vi "SVA 4MV6 T003 CCE.vi"() -> ()   [LabVIEW 2020]
panel:
  out "RGB":picture
  # "CEBALLOS CONDE  EMANUEL"
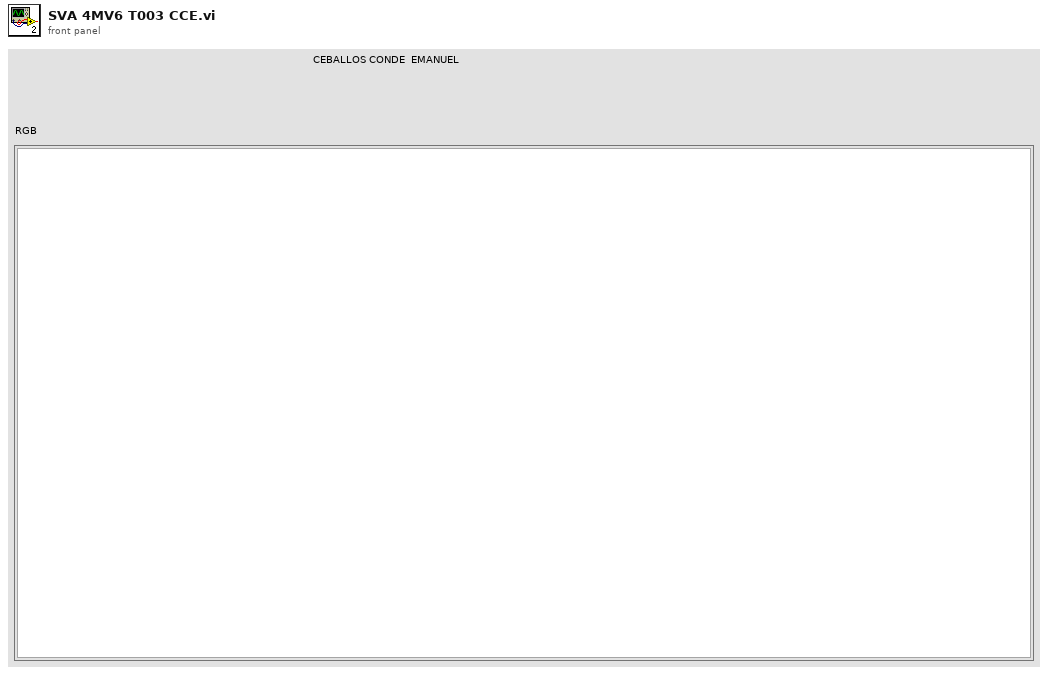
[diagram p1: front panel]
types:
  T1 = typedef "imagedata.ctl" = cluster{"image type":i32, "image depth":i32, "image":u8[], "mask":u8[], "colors":u32[], "Rectangle":cluster{"left":i16, "top":i16, "right":i16, "bottom":i16}}
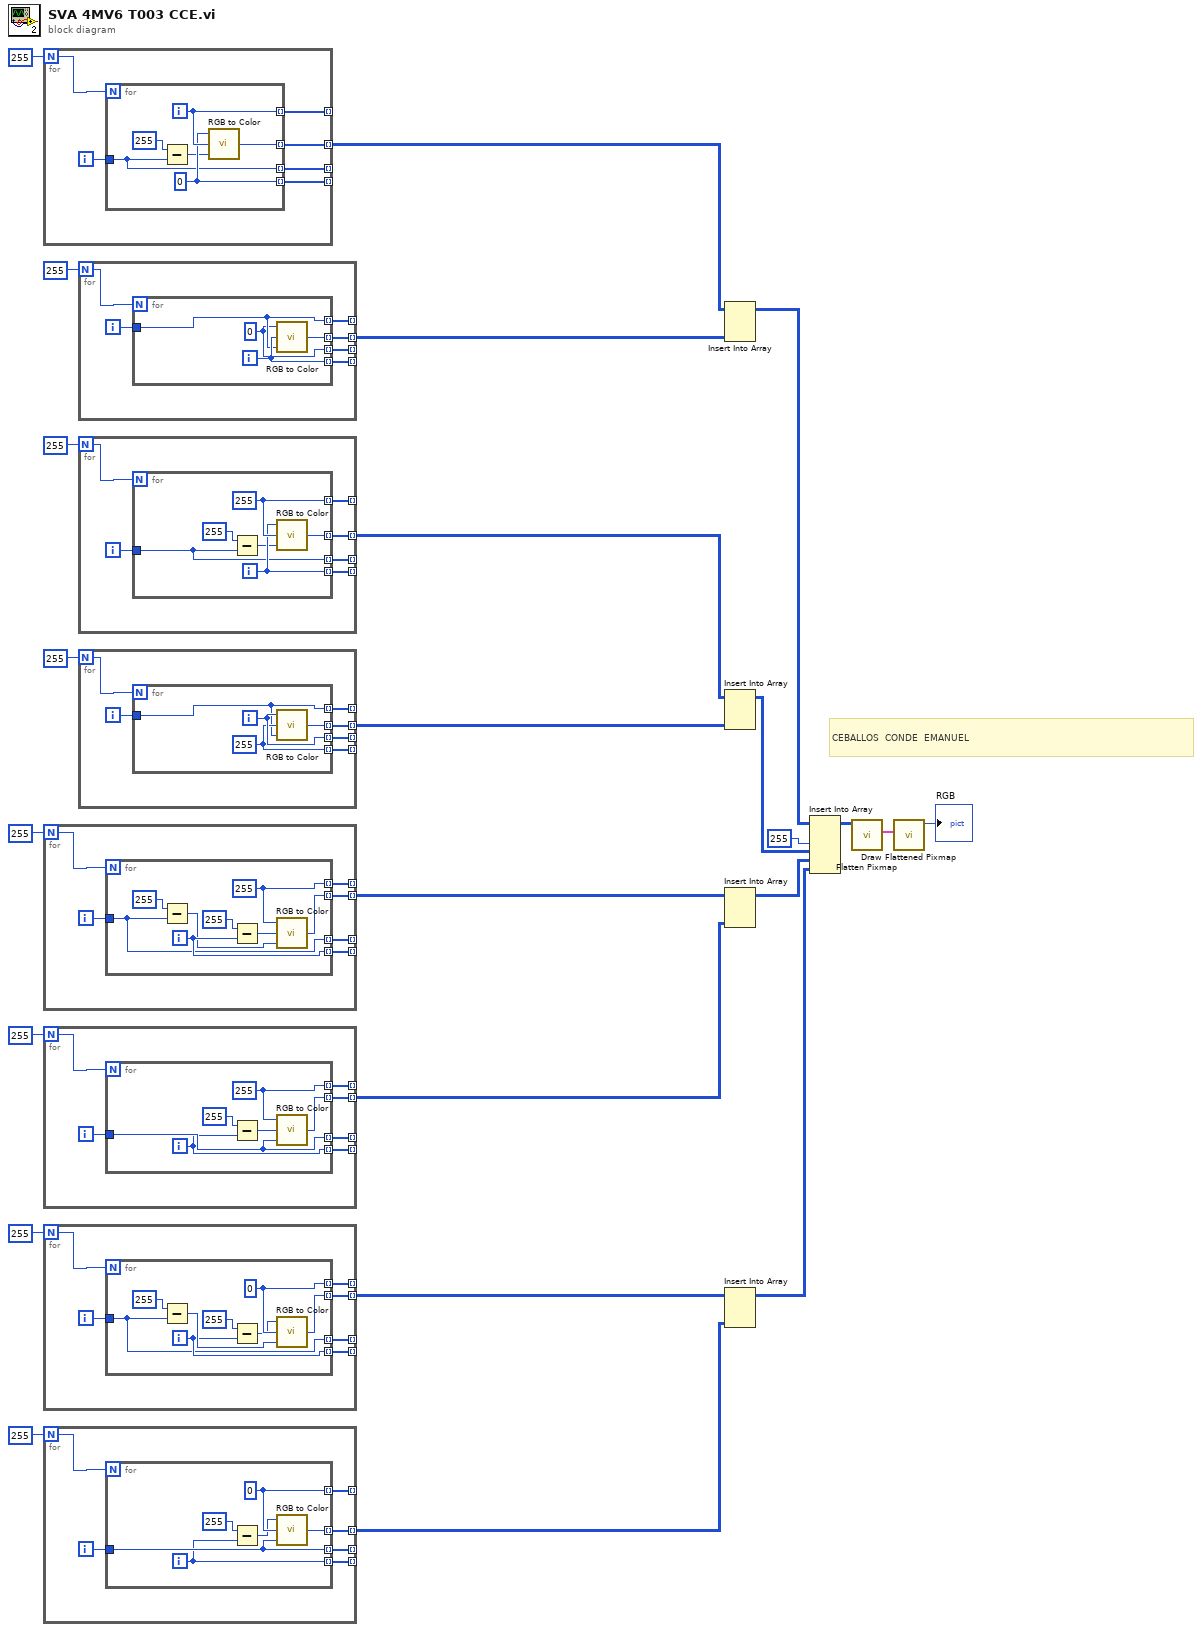
[diagram p0: block diagram]
diagram:
  # "CEBALLOS  CONDE  EMANUEL"
  n1 = for {
    N: 255 -> [w26]
    tunnel: [w30] -> _ mode=indexing
    tunnel: [w28] -> _ mode=indexing
    tunnel: [w27] -> _ mode=indexing
    tunnel: [w25] -> w4 mode=indexing
    i -> [w29]
    n2 = for {
      N: w26 -> [_]
      tunnel: [w35] -> w30 mode=indexing
      tunnel: w29 -> [w31]
      tunnel: [w31] -> w28 mode=indexing
      tunnel: [w34] -> w27 mode=indexing
      tunnel: [w36] -> w25 mode=indexing
      i -> [w35]
      w34 = 0
      n3 = Subtract(x=255, y=w31) -> (x-y=w32:i32)
      n4 = call <vilib>:"RGB to Color.vi"("B"=w32, "G"=w35, "R"=w34) -> ("Color"=w36:u32)
    }
  }
  n5 = for {
    N: 255 -> [w38]
    tunnel: [w42] -> _ mode=indexing
    tunnel: [w40] -> _ mode=indexing
    tunnel: [w39] -> _ mode=indexing
    tunnel: [w37] -> w14 mode=indexing
    i -> [w41]
    n6 = for {
      N: w38 -> [_]
      tunnel: [w48] -> w42 mode=indexing
      tunnel: w41 -> [w45]
      tunnel: [w45] -> w40 mode=indexing
      tunnel: [w44] -> w39 mode=indexing
      tunnel: [w50] -> w37 mode=indexing
      i -> [w48]
      w44 = 255
      n7 = Subtract(x=255, y=w45) -> (x-y=w46:i32)
      n8 = Subtract(x=255, y=w48) -> (x-y=w43:i32)
      n9 = call <vilib>:"RGB to Color.vi"("B"=w46, "G"=w43, "R"=w44) -> ("Color"=w50:u32)
    }
  }
  n10 = for {
    N: 255 -> [w52]
    tunnel: [w56] -> _ mode=indexing
    tunnel: [w54] -> _ mode=indexing
    tunnel: [w53] -> _ mode=indexing
    tunnel: [w51] -> w13 mode=indexing
    i -> [w55]
    n11 = for {
      N: w52 -> [_]
      tunnel: [w57] -> w56 mode=indexing
      tunnel: w55 -> [w60]
      tunnel: [w60] -> w54 mode=indexing
      tunnel: [w61] -> w53 mode=indexing
      tunnel: [w62] -> w51 mode=indexing
      i -> [w57]
      w61 = 255
      n12 = Subtract(x=255, y=w57) -> (x-y=w58:i32)
      n13 = call <vilib>:"RGB to Color.vi"("B"=w60, "G"=w58, "R"=w61) -> ("Color"=w62:u32)
    }
  }
  n14 = for {
    N: 255 -> [w64]
    tunnel: [w68] -> _ mode=indexing
    tunnel: [w66] -> _ mode=indexing
    tunnel: [w65] -> _ mode=indexing
    tunnel: [w63] -> w12 mode=indexing
    i -> [w67]
    n15 = for {
      N: w64 -> [_]
      tunnel: [w70] -> w68 mode=indexing
      tunnel: w67 -> [w69]
      tunnel: [w69] -> w66 mode=indexing
      tunnel: [w75] -> w65 mode=indexing
      tunnel: [w76] -> w63 mode=indexing
      i -> [w70]
      w75 = 0
      n16 = Subtract(x=255, y=w69) -> (x-y=w71:i32)
      n17 = Subtract(x=255, y=w70) -> (x-y=w73:i32)
      n18 = call <vilib>:"RGB to Color.vi"("B"=w71, "G"=w75, "R"=w73) -> ("Color"=w76:u32)
    }
  }
  n19 = for {
    N: 255 -> [w78]
    tunnel: [w82] -> _ mode=indexing
    tunnel: [w80] -> _ mode=indexing
    tunnel: [w79] -> _ mode=indexing
    tunnel: [w77] -> w3 mode=indexing
    i -> [w81]
    n20 = for {
      N: w78 -> [_]
      tunnel: [w83] -> w82 mode=indexing
      tunnel: w81 -> [w84]
      tunnel: [w84] -> w80 mode=indexing
      tunnel: [w87] -> w79 mode=indexing
      tunnel: [w88] -> w77 mode=indexing
      i -> [w83]
      w87 = 0
      n21 = Subtract(x=255, y=w83) -> (x-y=w85:i32)
      n22 = call <vilib>:"RGB to Color.vi"("B"=w84, "G"=w87, "R"=w85) -> ("Color"=w88:u32)
    }
  }
  n23 = for {
    N: 255 -> [w90]
    tunnel: [w94] -> _ mode=indexing
    tunnel: [w92] -> _ mode=indexing
    tunnel: [w91] -> _ mode=indexing
    tunnel: [w89] -> w5 mode=indexing
    i -> [w93]
    n24 = for {
      N: w90 -> [_]
      tunnel: [w97] -> w94 mode=indexing
      tunnel: w93 -> [w96]
      tunnel: [w96] -> w92 mode=indexing
      tunnel: [w95] -> w91 mode=indexing
      tunnel: [w98] -> w89 mode=indexing
      i -> [w97]
      w95 = 0
      n25 = call <vilib>:"RGB to Color.vi"("B"=w96, "G"=w97, "R"=w95) -> ("Color"=w98:u32)
    }
  }
  n26 = for {
    N: 255 -> [w100]
    tunnel: [w104] -> _ mode=indexing
    tunnel: [w102] -> _ mode=indexing
    tunnel: [w101] -> _ mode=indexing
    tunnel: [w99] -> w16 mode=indexing
    i -> [w103]
    n27 = for {
      N: w100 -> [_]
      tunnel: [w108] -> w104 mode=indexing
      tunnel: w103 -> [w105]
      tunnel: [w105] -> w102 mode=indexing
      tunnel: [w109] -> w101 mode=indexing
      tunnel: [w110] -> w99 mode=indexing
      i -> [w108]
      w109 = 255
      n28 = Subtract(x=255, y=w105) -> (x-y=w106:i32)
      n29 = call <vilib>:"RGB to Color.vi"("B"=w106, "G"=w109, "R"=w108) -> ("Color"=w110:u32)
    }
  }
  n30 = for {
    N: 255 -> [w112]
    tunnel: [w116] -> _ mode=indexing
    tunnel: [w114] -> _ mode=indexing
    tunnel: [w113] -> _ mode=indexing
    tunnel: [w111] -> w15 mode=indexing
    i -> [w115]
    n31 = for {
      N: w112 -> [_]
      tunnel: [w119] -> w116 mode=indexing
      tunnel: w115 -> [w117]
      tunnel: [w117] -> w114 mode=indexing
      tunnel: [w118] -> w113 mode=indexing
      tunnel: [w120] -> w111 mode=indexing
      i -> [w119]
      w118 = 255
      n32 = call <vilib>:"RGB to Color.vi"("B"=w117, "G"=w118, "R"=w119) -> ("Color"=w120:u32)
    }
  }
  n33 = Insert Into Array(array=w4, new element=w5) -> (w11:u32[][])  [unwired: 2 in]
  n34 = Insert Into Array(array=w16, new element=w15) -> (w10:u32[][])  [unwired: 2 in]
  n35 = Insert Into Array(array=w14, new element=w13) -> (w8:u32[][])  [unwired: 2 in]
  n36 = Insert Into Array(array=w12, new element=w3) -> (w7:u32[][])  [unwired: 2 in]
  n37 = Insert Into Array(array=w11, index (col)=255, new element #1=w10, new element #2=w8, new element #3=w7) -> (w9:u32[][])  [unwired: 1 in]
  n38 = call <vilib>:"Flatten Pixmap.vi"("24-bit pixmap"=w9) -> ("image data"=w18:T1)  [unwired: 10 in]
  n39 = call <vilib>:"Draw Flattened Pixmap.vi"("image data"=w18) -> ("new picture"=→"RGB":picture)  [unwired: 8 in]
